vi "Update From Result.vi"(8 "error in (no error)":errorcluster, 10 "Result Row":refnum<class "Result Row.lvclass">, 11 "Long Class Name Entity Example in":refnum<class "Long Class Name Entity Example.lvclass">) -> (0 "error out":errorcluster, 3 "Long Class Name Entity Example out":refnum<class "Long Class Name Entity Example.lvclass">)   [LabVIEW 2022 SP3]
uses:
  Long Class Name Entity Example.lvclass
  Conditum/Result Row/Result Row.lvclass
  Long Class Name Entity Example.lvclass/Long Class Name Entity Example.ctl
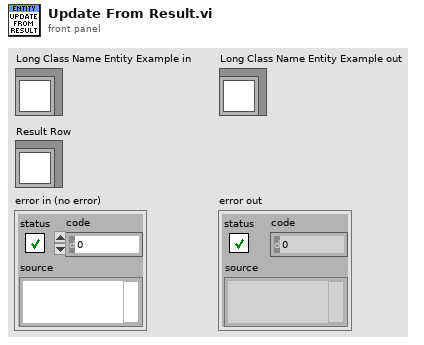
[diagram p1: front panel]
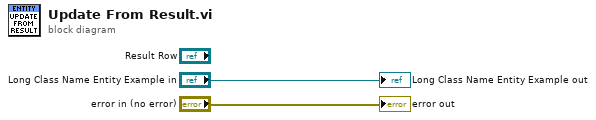
[diagram p0: block diagram]
diagram:
  "error out" <- "error in (no error)"
  "Long Class Name Entity Example out" <- "Long Class Name Entity Example in"
